vi "str to boolean.vi"(2 "String":string) -> (6 "Boolean":bool)   [LabVIEW 2013]
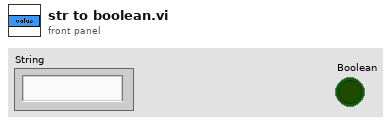
[diagram p1: front panel]
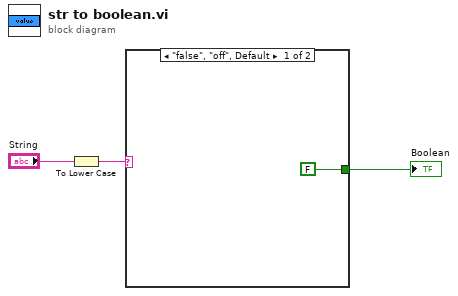
[diagram p0: block diagram]
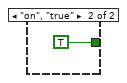
[diagram p2: hidden frame]
diagram:
  n1 = To Lower Case(string="String") -> (all lower case string=w2:string)
  n2 = case shown="\"false\", \"off\", Default" w2 {
    tunnel: [FALSE TRUE] -> w1
    frame "false", "off", Default {
    }
    frame "on", "true" {
    }
  }
  "Boolean" <- w1
